vi "1 - MQTT_Q_Example.vi"() -> ()   [LabVIEW 2015]
uses:
  source/MQTT_Q.lvclass
panel:
  out "Topic Received":string
  in  "Send":bool
  out "String Received":string
  in  "String to send":string
  in  "Exit":bool
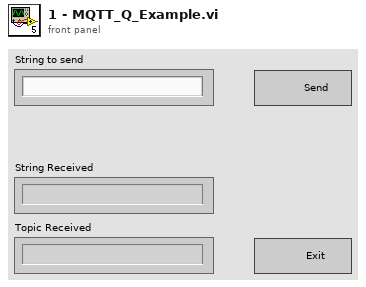
[diagram p1: front panel]
types:
  T1 = cluster{"IP address":string, "Port":u16, "Client ID":string}
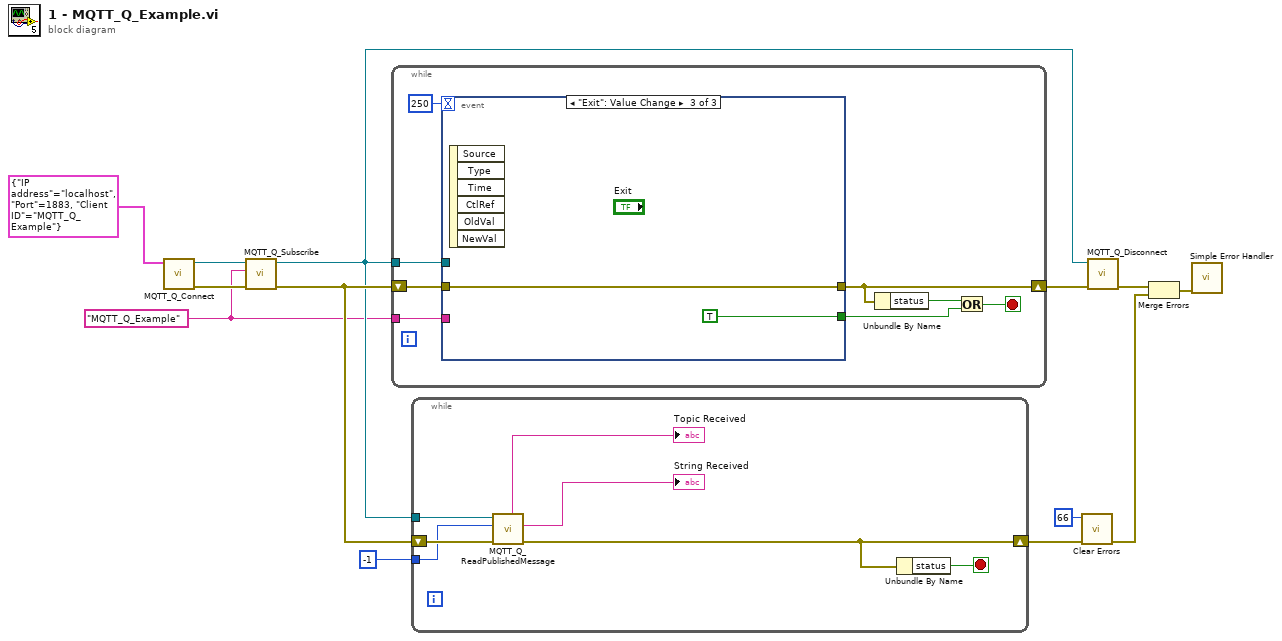
[diagram p0: block diagram]
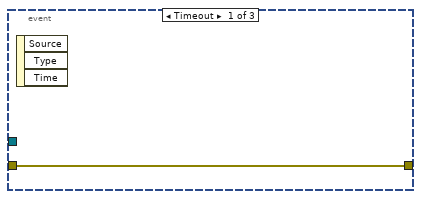
[diagram p2: hidden frame]
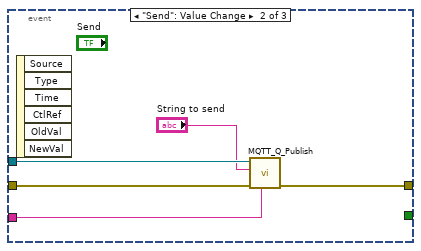
[diagram p3: hidden frame]
diagram:
  w1 = "MQTT_Q_Example" ("Topic")
  n1 = call "MQTT_Q_Connect.vi"("MQTT Broker & Client ID"=T1 {"IP address"="localhost", "Port"=1883, "Client ID"="MQTT_Q_Example"}) -> ("error out"=w12:errorcluster, "MQTT_Q Out"=w11:refnum<class "MQTT_Q.lvclass">)  [unwired: 9 in]
  n2 = call "MQTT_Q_Subscribe.vi"("error in (no error)"=w12, "Topic"=w1, "MQTT_Q In"=w11) -> ("error out"=w10:errorcluster, "MQTT_Q Out"=w9:refnum<class "MQTT_Q.lvclass">)  [unwired: 6 in, 1 out]
  n3 = while {
    shift-right: [w17] -> w7
    shift-left: w10 -> [w21]
    tunnel: w9 -> [w20]
    tunnel: w1 -> [w19]
    stop <- w14 stop-if-true
    n4 = event shown="[2] \"Exit\": Value Change" {
      selector: _ -> [_ _ _]
      dyn-events: _ -> [_ _ _]
      timeout: 250 -> [_ _ _]
      tunnel: w21 -> [w22 w27 w29]
      tunnel: w20 -> [_ w25 _]
      tunnel: [w22 w26 w29] -> w17
      tunnel: w19 -> [_ w24 _]
      tunnel: [_ _ TRUE] -> w15
      event Timeout {
        n5 = event-data() -> ()  [unwired: 1 in, 3 out]
      }
      event "Send": Value Change {
        n6 = event-data() -> ()  [unwired: 1 in, 6 out]
        n7 = call "MQTT_Q_Publish.vi"("Topic"=w24, "error in"=w27, "Message"="String to send", "MQTT_Q In"=w25) -> ("error out"=w26:errorcluster)  [unwired: 6 in, 1 out]
      }
      event "Exit": Value Change {
        n8 = event-data() -> ()  [unwired: 1 in, 6 out]
      }
    }
    n9 = Unbundle By Name(w17) -> ("status"=w16:bool)
    n10 = Or(x=w16, y=w15) -> (x .or. y?=w14:bool)
  }
  n11 = while {
    shift-right: [w35] -> w4
    shift-left: w10 -> [w36]
    tunnel: w9 -> [w34]
    tunnel: -1 ("timeout in ms (-1)") -> [w33]
    stop <- w32 stop-if-true
    n12 = call "MQTT_Q_ReadPublishedMessage.vi"("error in (no error)"=w36, "timeout ms (25000)"=w33, "MQTT_Q In"=w34) -> ("error out"=w35:errorcluster, "Message"=→"String Received":string, "Topic"=→"Topic Received":string)  [unwired: 4 in, 2 out]
    n13 = Unbundle By Name(w35) -> ("status"=w32:bool)
  }
  n14 = call <vilib>:"Clear Errors.vi"("error in (no error)"=w4, "specific error code to clear (0: all)"=66) -> ("error out"=w3:errorcluster)  [unwired: 4 in, 1 out]
  n15 = call "MQTT_Q_Disconnect.vi"("error in (no error)"=w7, "MQTT_Q In"=w9) -> ("error out"=w6:errorcluster)  [unwired: 9 in]
  n16 = Merge Errors(w6, w3) -> (w5:errorcluster)
  n17 = call <vilib>:"Simple Error Handler.vi"("error in (no error)"=w5) -> ()  [unwired: 4 in, 5 out]
